vi "LabVIEW中的高等数学运算.vi"() -> ()   [LabVIEW 2018]
uses:
  <vilib>/Analysis/polynomials.llb/Polynomial Roots (DBL).vi
  <vilib>/Analysis/NI_AALBase.lvlib
  <vilib>/Analysis/NI_AALPro.lvlib
panel:
  out "Roots":cdb[](array[numeric]) caption="根"
  out "Polynomial Coefficients":dbl[](array[numeric]) caption="多项式系数"
  out "variance":dbl caption="方差" format="%0.2f"
  out "standard deviation":dbl caption="标准差" format="%0.2f"
  out "mean":dbl caption="均值" format="%0.2f"
  out "问题1":dbl[](array[numeric])
  # "问题2"
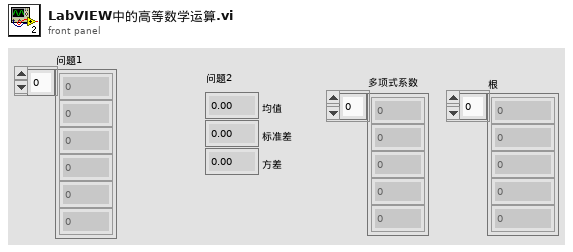
[diagram p1: front panel]
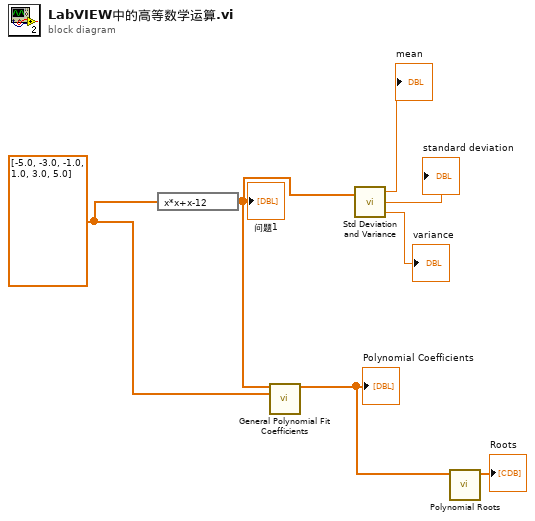
[diagram p0: block diagram]
diagram:
  w4 = dbl[] [-5.0, -3.0, -1.0, 1.0, 3.0, 5.0]
  n1 = expression code="x*x+x-12"(w4) -> (w3:dbl[])
  "问题1" <- w3
  n2 = call <vilib>:"General Polynomial Fit Coefficients.vi"("Y"=w3, "X"=w4) -> ("Polynomial Coefficients"=w2:dbl[])  [unwired: 12 in, 1 out]
  "Polynomial Coefficients" <- w2
  n3 = call <vilib>:"Std Deviation and Variance.vi"("X"=w3) -> ("mean"=→"mean":dbl, "standard deviation"=→"standard deviation":dbl, "variance"=→"variance":dbl)  [unwired: 1 in]
  n4 = call-poly <vilib>:"Polynomial Roots.vi"("P(x)"=w2) -> ("Roots"=→"Roots":cdb[])  [unwired: 9 in, 1 out]
